vi "Feather Constructor.vi"(8 "error in (no error)":errorcluster, 9 "y vector":dbl[](array[numeric]), 10 "x vector":dbl[](array[numeric]), 11 "2D Feather Datatype.lvclass in":refnum<class "2D Feather Datatype.lvclass">) -> (0 "error out":errorcluster, 3 "2D Feather Datatype.lvclass out":refnum<class "2D Feather Datatype.lvclass">)   [LabVIEW 2020, in "2D Feather Datatype.lvclass"]
uses:
  <vilib>/Math Plots/2D Math Plots/2D Feather/2D Feather Datatype/2D Feather Datatype.lvclass
  <vilib>/Math Plots/2D Math Plots/2D Feather/2D Feather Datatype/2D Feather Datatype.lvclass/2D Feather Datatype.ctl
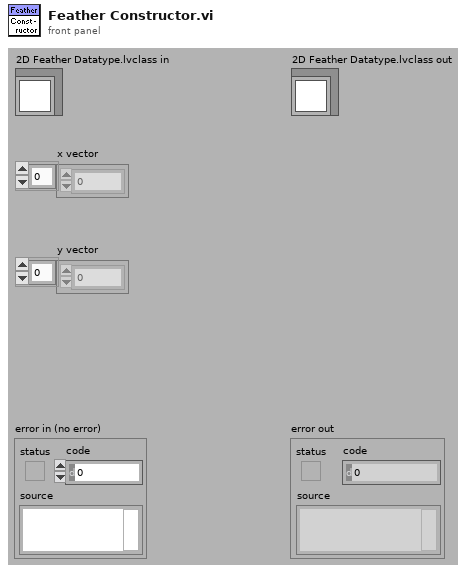
[diagram p1: front panel]
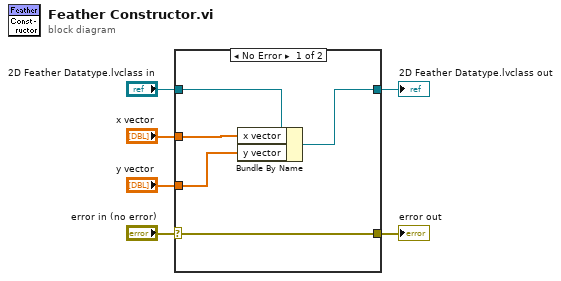
[diagram p0: block diagram]
diagram:
  n1 = case shown="No Error" "error in (no error)" {
    selector: "error in (no error)" -> [w11 w13]
    tunnel: [w11 w13] -> w2
    tunnel: "x vector" -> [w9 _]
    tunnel: "y vector" -> [w8 _]
    tunnel: "2D Feather Datatype.lvclass in" -> [w10 w12]
    tunnel: [w7 w12] -> w6
    frame No Error {
      n2 = Bundle By Name(cluster=w10, "x vector"=w9, "y vector"=w8) -> (w7:refnum<class "2D Feather Datatype.lvclass">)
    }
    frame Error {
    }
  }
  "error out" <- w2
  "2D Feather Datatype.lvclass out" <- w6
